vi "Digital Serial Configuration Popup.vi"() -> ()   [LabVIEW 2021, in "Audio Popup UI.lvlib"]
uses:
  Audio Popup UI.lvlib
  controls/digital audio protocol/digital audio protocol settings.ctl
  <vilib>/PDM Acquisition Toolkit/shared/controls/PCM Data Justification.ctl
  <vilib>/PDM Acquisition Toolkit/shared/controls/PCM Bit Endianness.ctl
  <vilib>/PDM Acquisition Toolkit/shared/controls/Digital Edge.ctl
  <vilib>/PDM Acquisition Toolkit/host/Classes/Session/Controls/Logic Levels.ctl
  <vilib>/PDM Acquisition Toolkit/shared/PDM Shared.lvlib
  <vilib>/PDM Acquisition Toolkit/host/Classes/Session/DecoderSession.lvclass
  controls/digital audio protocol/digital audio protocol controls.lvlib
panel:
  in  "channel 0 offset":u32=1
  in  "Save":bool
  in  "Configuration File":path
  in  "logic level":enum32{"3.3 V", "1.8 V", "1.2 V"}(ring) caption="Logic level"
  in  "master clock rate":dbl=12288000.0 caption="Master clock rate" format="%#_6pHz"
  out "Bit clock rate":dbl=3072000.0 format="%#_6pHz"
  in  "number of channels":u32=2 caption="Number of channels"
  in  "TDM":bool
  in  "RJ":bool
  in  "LJ":bool
  in  "I2S":bool
  in  "bit clock edge sync":enum32{"Rising", "Falling"}(ring)=enum."Falling" caption="Bit clock edge sync"
  in  "frame clock rate":dbl=48000.0 caption="Frame clock rate" format="%#_6pHz"
  in  "data justification":enum32{"Left Justified", "Right Justified"}(ring) caption="Data justification"
  in  "endianness":enum32{"MSB First", "LSB First"}(ring) caption="Endianness"
  in  "bit depth":u32=24 caption="Bit depth"
  in  "channel length":u32=32 caption="Channel length"
  in  "frame sync edge for channel 0":enum32{"Rising", "Falling"}(ring)=enum."Falling" caption="Frame sync edge for Channel 0"
  # "Audio Protocol"
  # "Clock Settings"
  # "Signal Level"
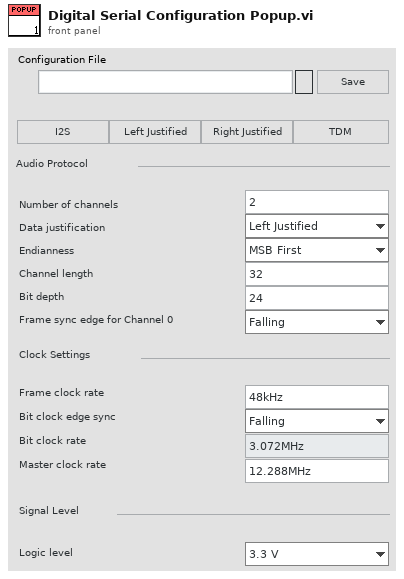
[diagram p1: front panel]
types:
  T1 = typedef "digital audio protocol controls.lvlib/digital audio protocol settings.ctl" = cluster{"number of channels":u32, "data justification":T2, "endianness":T3, "channel length":u32, "bit depth":u32, "frame clock rate":dbl, "bit clock edge sync":T4, "master clock rate":dbl, "Logic Level":T5, "frame sync edge for channel 0":T4, "Channel 0 Offset":u32}
  T2 = typedef "PDM Shared.lvlib/PCM Data Justification.ctl" = enum16{"Left Justified", "Right Justified"}
  T3 = typedef "PDM Shared.lvlib/PCM Bit Endianness.ctl" = enum16{"MSB First", "LSB First"}
  T4 = typedef "PDM Shared.lvlib/Digital Edge.ctl" = enum8{"Rising", "Falling"}
  T5 = typedef "PDM Acquisition Class Library.lvlib/DecoderSession.lvclass/Logic Levels.ctl" = enum16{"3.3 V", "1.8 V", "1.2 V"}
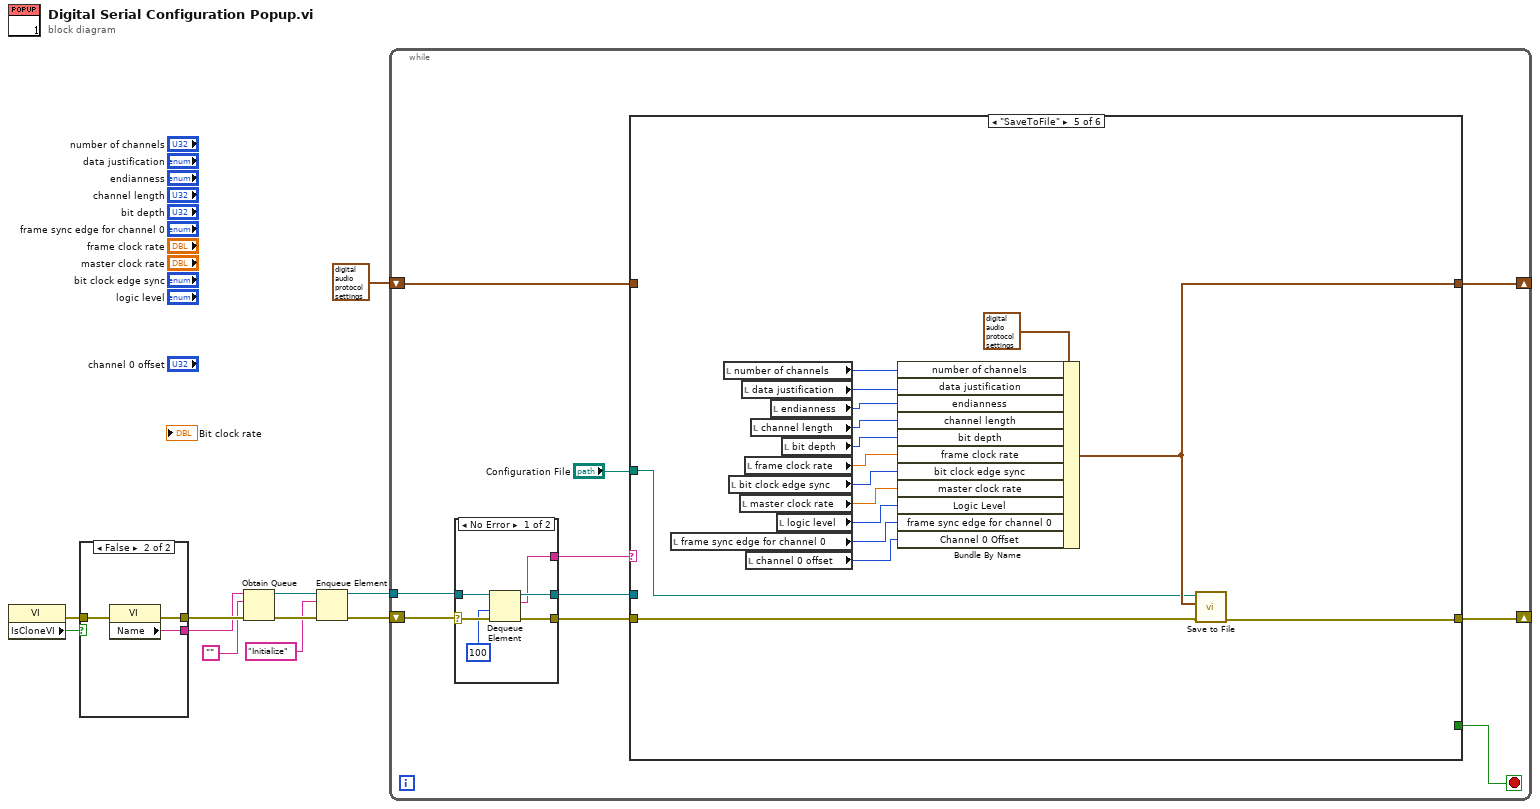
[diagram p0: block diagram]
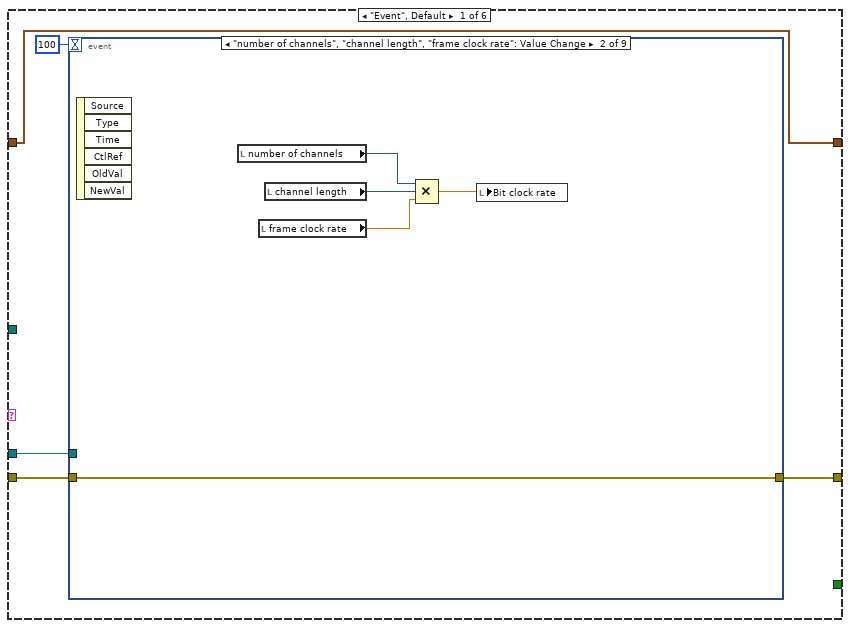
[diagram p2: hidden frame]
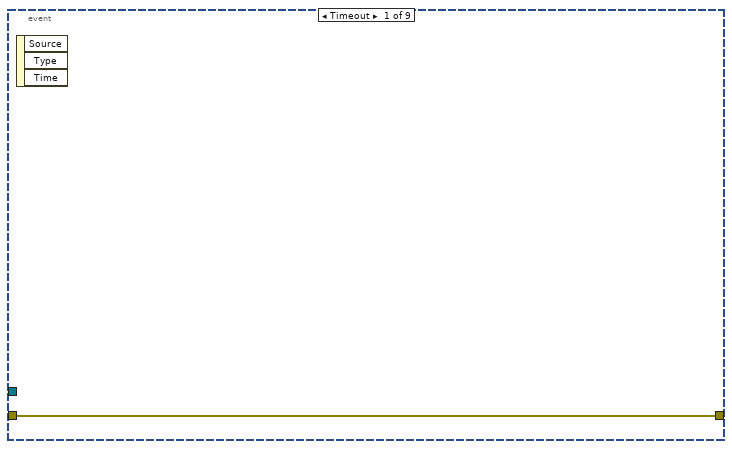
[diagram p3: hidden frame]
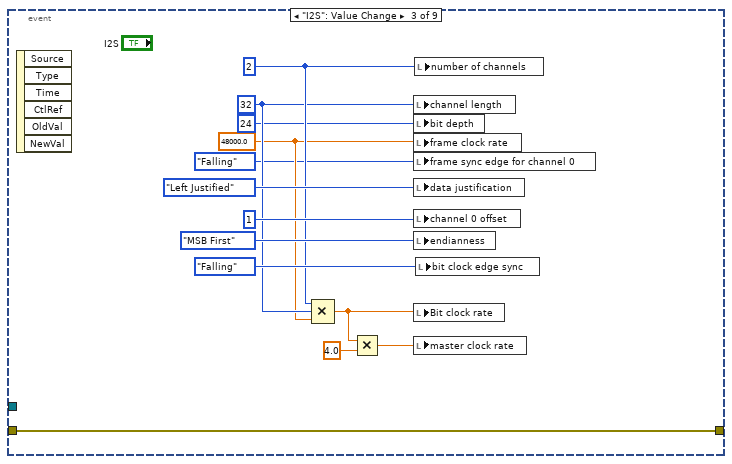
[diagram p4: hidden frame]
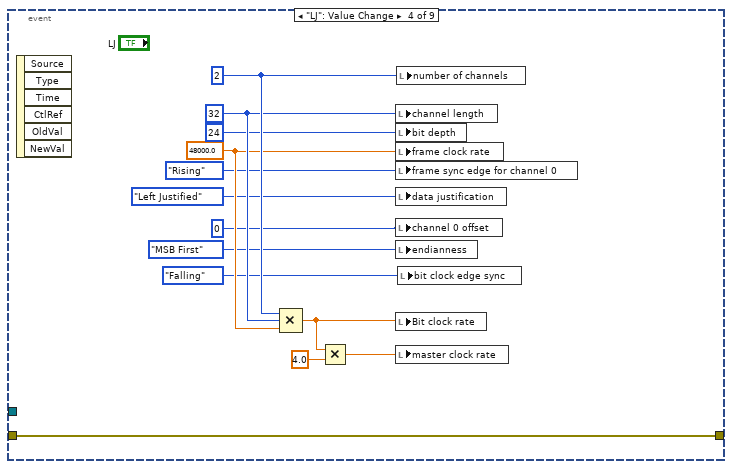
[diagram p5: hidden frame]
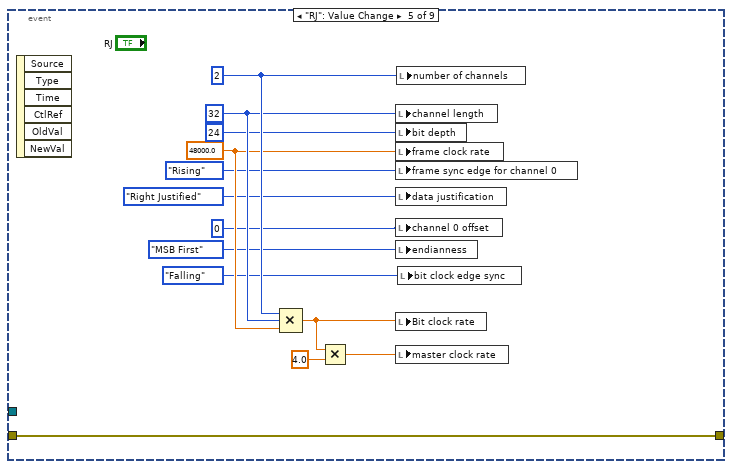
[diagram p6: hidden frame]
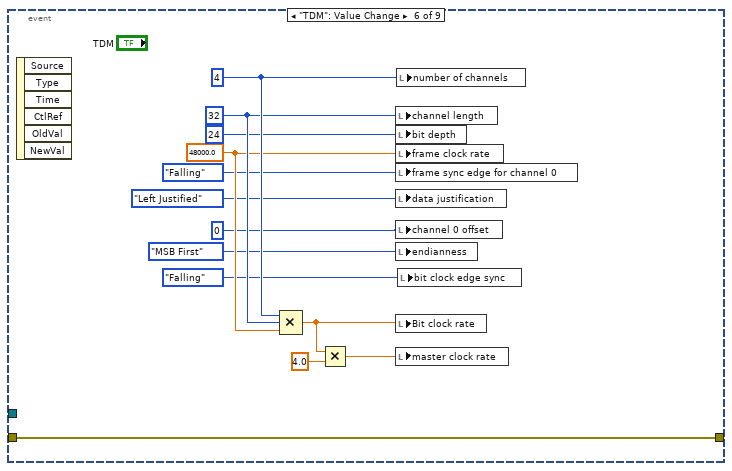
[diagram p7: hidden frame]
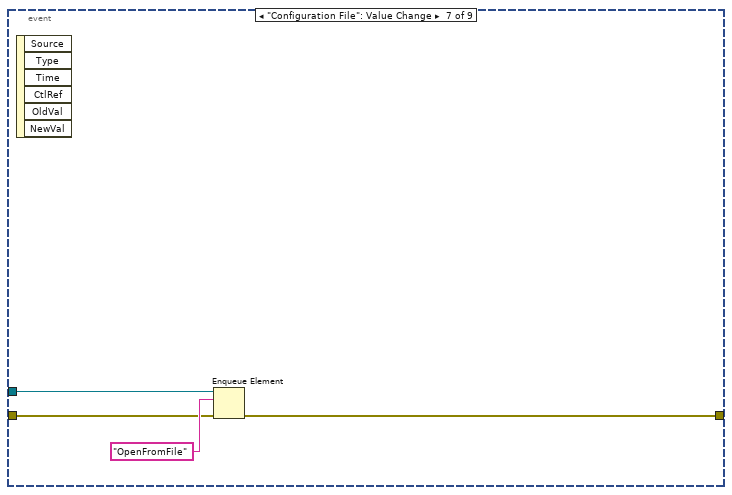
[diagram p8: hidden frame]
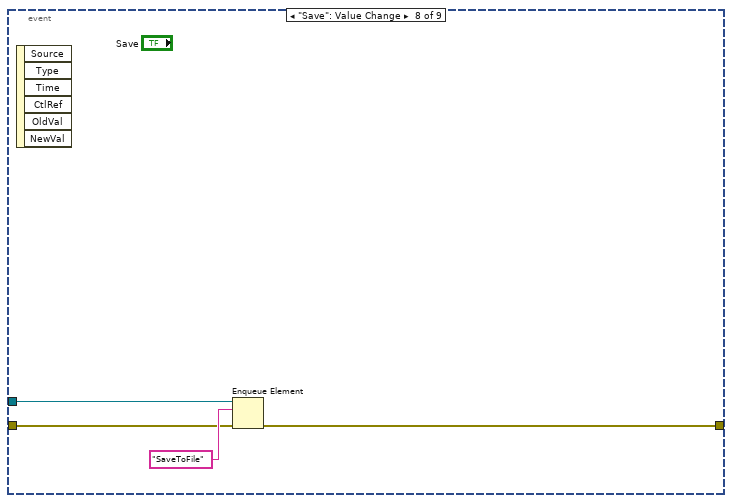
[diagram p9: hidden frame]
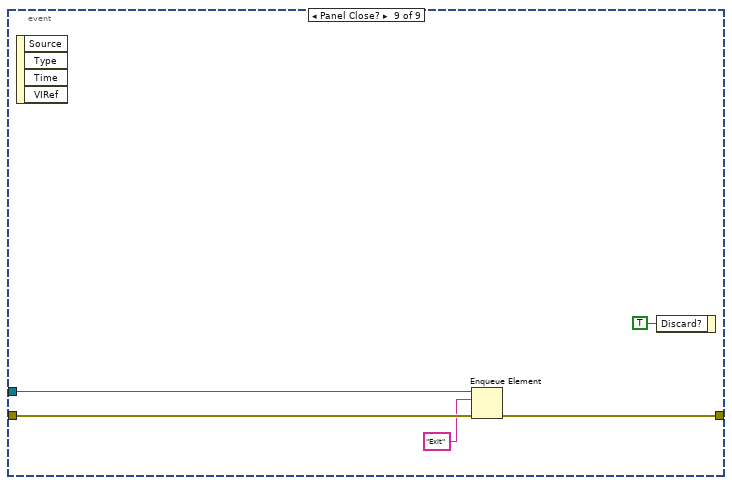
[diagram p10: hidden frame]
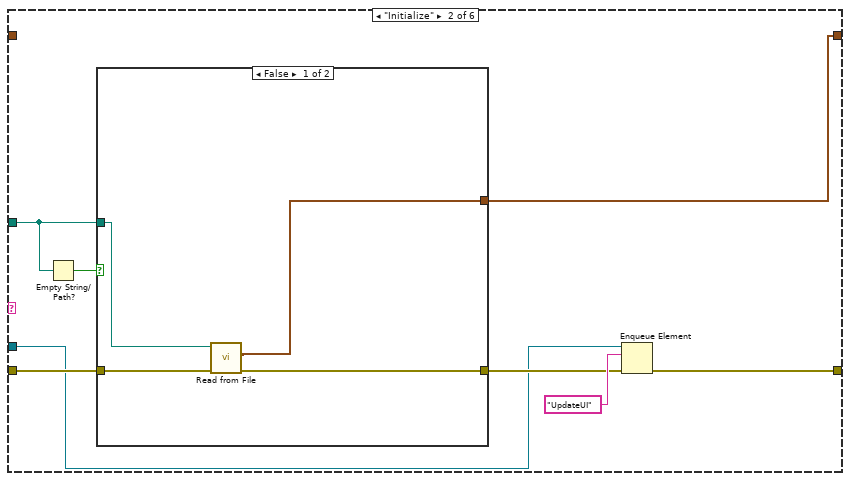
[diagram p11: hidden frame]
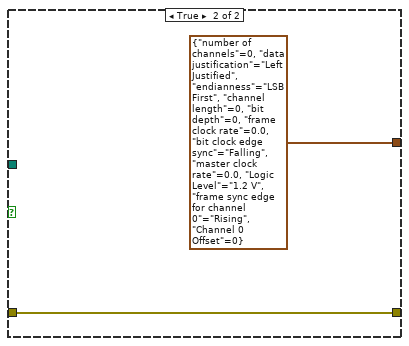
[diagram p12: hidden frame]
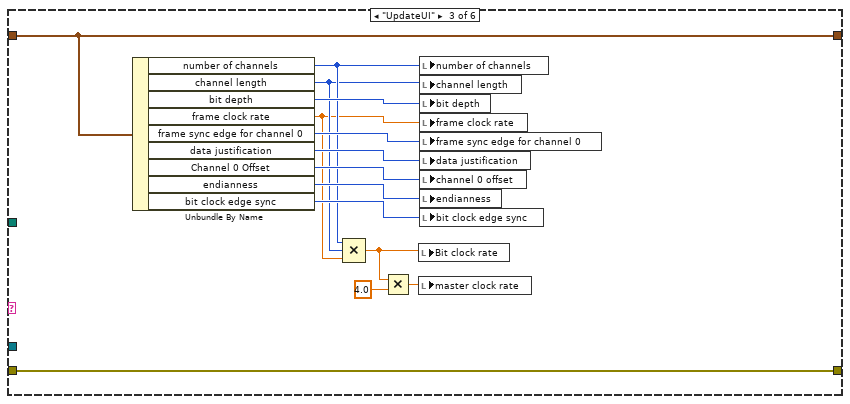
[diagram p13: hidden frame]
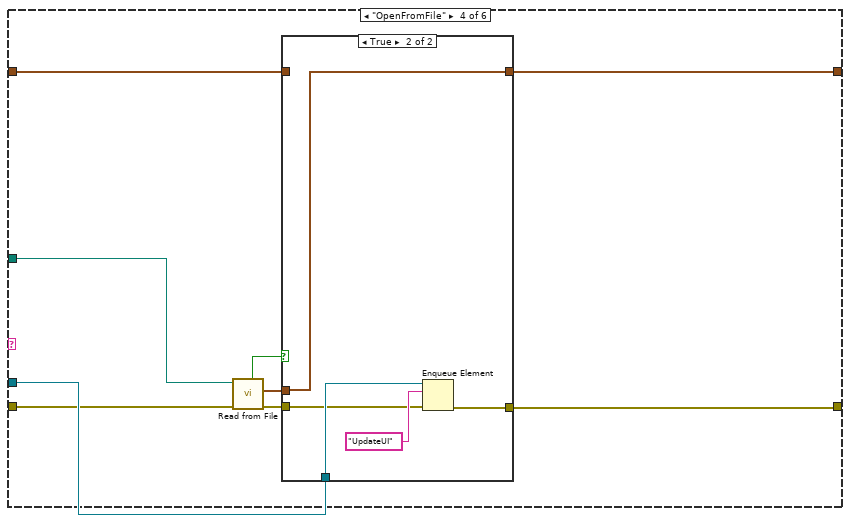
[diagram p14: hidden frame]
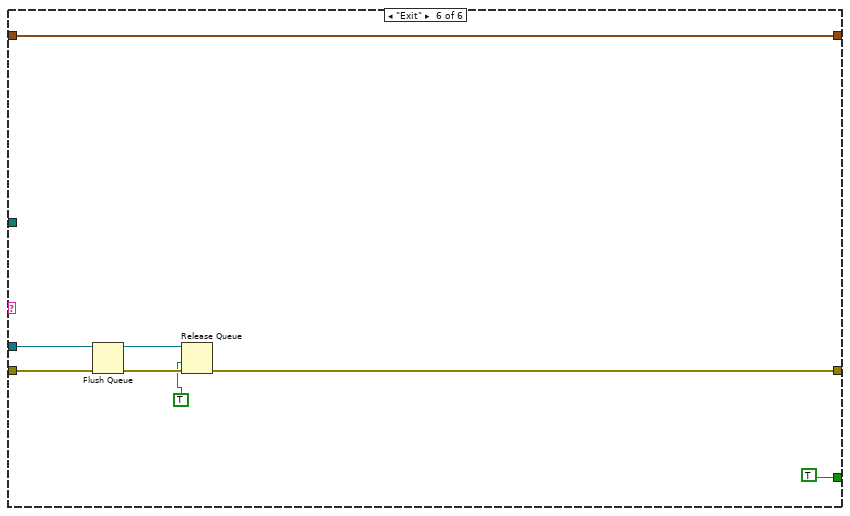
[diagram p16: hidden frame]
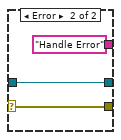
[diagram p17: hidden frame]
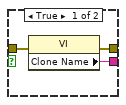
[diagram p18: hidden frame]
diagram:
  n1 = property class="VI"() -> (error out=w4:errorcluster, "IsCloneVI"=w5:bool)  [unwired: 2 in, 1 out]
  n2 = case shown="False" w5 {
    tunnel: [w14 w17] -> w11
    tunnel: [w13 w16] -> w10
    tunnel: w4 -> [w12 w15]
    frame True {
      n3 = property class="VI"(error in=w12) -> (error out=w14:errorcluster, "Clone Name"=w13:string)  [unwired: 1 in, 1 out]
    }
    frame False {
      n4 = property class="VI"(error in=w15) -> (error out=w17:errorcluster, "Name"=w16:string)  [unwired: 1 in, 1 out]
    }
  }
  n5 = Obtain Queue(name (unnamed)=w10, element data type="", error in (no error)=w11) -> (queue out=w8:refnum<queue>, error out=w9:errorcluster)  [unwired: 2 in, 1 out]
  n6 = Enqueue Element(queue=w8, element="Initialize", error in (no error)=w9) -> (queue out=w2:refnum<queue>, error out=w3:errorcluster)  [unwired: 1 in, 1 out]
  n7 = while {
    tunnel: w2 -> [w26]
    shift-right: [w22] -> _
    shift-left: w3 -> [w27]
    shift-right: [w19] -> _
    shift-left: T1 {"number of channels"=0, "data justification"=enum."Left Justified", "endianness"=enum."LSB First", "channel length"=0, "bit depth"=0, "frame clock rate"=0.0, "bit clock edge sync"=enum."Falling", "master clock rate"=0.0, "Logic Level"=enum."1.2 V", "frame sync edge for channel 0"=enum."Rising", "Channel 0 Offset"=0} ("digital audio protocol settings") -> [w20]
    stop <- w21 stop-if-true
    n8 = case shown="No Error" w27 {
      selector: w27 -> [w177 w180]
      tunnel: [w176 w180] -> w23
      tunnel: w26 -> [w175 w179]
      tunnel: [w174 w179] -> w24
      tunnel: [w173 "Handle Error"] -> w25
      frame No Error {
        n9 = Dequeue Element(queue=w175, timeout in ms (-1)=100, error in (no error)=w177) -> (queue out=w174:refnum<queue>, element=w173:string, error out=w176:errorcluster)  [unwired: 1 out]
      }
      frame Error {
      }
    }
    n10 = case shown="\"SaveToFile\"" w25 {
      tunnel: w24 -> [w30 w104 _ w140 _ w167]
      tunnel: w23 -> [w31 w111 w131 w137 w151 w168]
      tunnel: [w29 w105 w131 w139 w150 w165] -> w22
      tunnel: [_ _ _ _ _ TRUE] -> w21
      tunnel: w20 -> [w28 _ w130 w134 _ w164]
      tunnel: [w28 w108 w130 w133 w149 w164] -> w19
      tunnel: "Configuration File" -> [_ w109 _ w138 w148 _]
      frame "Event", Default {
        n11 = event shown="[1] \"number of channels\", \"channel length\", \"frame clock rate\": Value Change" {
          selector: _ -> [_ _ _ _ _ _ _ _ _]
          dyn-events: _ -> [_ _ _ _ _ _ _ _ _]
          timeout: 100 -> [_ _ _ _ _ _ _ _ _]
          tunnel: w31 -> [w33 w34 w39 w52 w65 w78 w93 w97 w102]
          tunnel: w30 -> [_ _ _ _ _ _ w92 w96 w101]
          tunnel: [w33 w34 w39 w52 w65 w78 w91 w95 w100] -> w29
          event Timeout {
            n12 = event-data() -> ()  [unwired: 1 in, 3 out]
          }
          event "number of channels", "channel length", "frame clock rate": Value Change {
            n13 = event-data() -> ()  [unwired: 1 in, 6 out]
            n14 = local read "number of channels"() -> (w36:u32)
            n15 = local read "frame clock rate"() -> (w35:dbl)
            n16 = local read "channel length"() -> (w37:u32)
            n17 = Compound Arithmetic op=MULTIPLY(w36, w37, w35) -> (w38:dbl)
            n18 = local write "Bit clock rate"(w38) -> ()
          }
          event "I2S": Value Change {
            w42 = 48000.0 ("Frame Clock Rate")
            w43 = u32 32 ("Channel Length")
            w44 = u32 2 ("Number of Channels")
            n19 = event-data() -> ()  [unwired: 1 in, 6 out]
            n20 = Compound Arithmetic op=MULTIPLY(w44, w43, w42) -> (w50:dbl)
            n21 = Multiply(x=w50, y=4.0) -> (x*y=w49:dbl)
            n22 = local write "channel length"(w43) -> ()
            n23 = local write "bit depth"(u32 24 ("Bit Depth")) -> ()
            n24 = local write "frame clock rate"(w42) -> ()
            n25 = local write "frame sync edge for channel 0"(enum32{"Rising", "Falling"}."Falling" ("bit clock edge sync")) -> ()
            n26 = local write "data justification"(enum32{"Left Justified", "Right Justified"}."Left Justified" ("data justification")) -> ()
            n27 = local write "channel 0 offset"(u32 1 ("Channel 0 Offset")) -> ()
            n28 = local write "endianness"(enum32{"MSB First", "LSB First"}."MSB First" ("endianness")) -> ()
            n29 = local write "Bit clock rate"(w50) -> ()
            n30 = local write "master clock rate"(w49) -> ()
            n31 = local write "number of channels"(w44) -> ()
            n32 = local write "bit clock edge sync"(enum32{"Rising", "Falling"}."Falling" ("frame sync edge for channel 0")) -> ()
          }
          event "LJ": Value Change {
            w60 = 48000.0 ("Frame Clock Rate")
            w62 = u32 32 ("Channel Length")
            w63 = u32 2 ("Number of Channels")
            n33 = event-data() -> ()  [unwired: 1 in, 6 out]
            n34 = Compound Arithmetic op=MULTIPLY(w63, w62, w60) -> (w54:dbl)
            n35 = Multiply(x=w54, y=4.0) -> (x*y=w53:dbl)
            n36 = local write "channel length"(w62) -> ()
            n37 = local write "bit depth"(u32 24 ("Bit Depth")) -> ()
            n38 = local write "frame clock rate"(w60) -> ()
            n39 = local write "frame sync edge for channel 0"(enum32{"Rising", "Falling"}."Rising" ("bit clock edge sync")) -> ()
            n40 = local write "data justification"(enum32{"Left Justified", "Right Justified"}."Left Justified" ("data justification")) -> ()
            n41 = local write "channel 0 offset"(u32 0 ("Channel 0 Offset")) -> ()
            n42 = local write "endianness"(enum32{"MSB First", "LSB First"}."MSB First" ("endianness")) -> ()
            n43 = local write "Bit clock rate"(w54) -> ()
            n44 = local write "master clock rate"(w53) -> ()
            n45 = local write "number of channels"(w63) -> ()
            n46 = local write "bit clock edge sync"(enum32{"Rising", "Falling"}."Falling" ("frame sync edge for channel 0")) -> ()
          }
          event "RJ": Value Change {
            w73 = 48000.0 ("Frame Clock Rate")
            w75 = u32 32 ("Channel Length")
            w76 = u32 2 ("Number of Channels")
            n47 = event-data() -> ()  [unwired: 1 in, 6 out]
            n48 = Compound Arithmetic op=MULTIPLY(w76, w75, w73) -> (w67:dbl)
            n49 = Multiply(x=w67, y=4.0) -> (x*y=w66:dbl)
            n50 = local write "channel length"(w75) -> ()
            n51 = local write "bit depth"(u32 24 ("Bit Depth")) -> ()
            n52 = local write "frame clock rate"(w73) -> ()
            n53 = local write "frame sync edge for channel 0"(enum32{"Rising", "Falling"}."Rising" ("bit clock edge sync")) -> ()
            n54 = local write "data justification"(enum32{"Left Justified", "Right Justified"}."Right Justified" ("data justification")) -> ()
            n55 = local write "channel 0 offset"(u32 0 ("Channel 0 Offset")) -> ()
            n56 = local write "endianness"(enum32{"MSB First", "LSB First"}."MSB First" ("endianness")) -> ()
            n57 = local write "Bit clock rate"(w67) -> ()
            n58 = local write "master clock rate"(w66) -> ()
            n59 = local write "number of channels"(w76) -> ()
            n60 = local write "bit clock edge sync"(enum32{"Rising", "Falling"}."Falling" ("frame sync edge for channel 0")) -> ()
          }
          event "TDM": Value Change {
            w86 = 48000.0 ("Frame Clock Rate")
            w88 = u32 32 ("Channel Length")
            w89 = u32 4 ("Number of Channels")
            n61 = event-data() -> ()  [unwired: 1 in, 6 out]
            n62 = Compound Arithmetic op=MULTIPLY(w89, w88, w86) -> (w80:dbl)
            n63 = Multiply(x=w80, y=4.0) -> (x*y=w79:dbl)
            n64 = local write "channel length"(w88) -> ()
            n65 = local write "bit depth"(u32 24 ("Bit Depth")) -> ()
            n66 = local write "frame clock rate"(w86) -> ()
            n67 = local write "frame sync edge for channel 0"(enum32{"Rising", "Falling"}."Falling" ("bit clock edge sync")) -> ()
            n68 = local write "data justification"(enum32{"Left Justified", "Right Justified"}."Left Justified" ("data justification")) -> ()
            n69 = local write "channel 0 offset"(u32 0 ("Channel 0 Offset")) -> ()
            n70 = local write "endianness"(enum32{"MSB First", "LSB First"}."MSB First" ("endianness")) -> ()
            n71 = local write "Bit clock rate"(w80) -> ()
            n72 = local write "master clock rate"(w79) -> ()
            n73 = local write "number of channels"(w89) -> ()
            n74 = local write "bit clock edge sync"(enum32{"Rising", "Falling"}."Falling" ("frame sync edge for channel 0")) -> ()
          }
          event "Configuration File": Value Change {
            n75 = event-data() -> ()  [unwired: 1 in, 6 out]
            n76 = Enqueue Element(queue=w92, element="OpenFromFile", error in (no error)=w93) -> (error out=w91:errorcluster)  [unwired: 1 in, 2 out]
          }
          event "Save": Value Change {
            n77 = event-data() -> ()  [unwired: 1 in, 6 out]
            n78 = Enqueue Element(queue=w96, element="SaveToFile", error in (no error)=w97) -> (error out=w95:errorcluster)  [unwired: 1 in, 2 out]
          }
          event Panel Close? {
            n79 = event-data() -> ()  [unwired: 1 in, 4 out]
            n80 = Enqueue Element(queue=w101, element="Exit", error in (no error)=w102) -> (error out=w100:errorcluster)  [unwired: 1 in, 2 out]
            n81 = event-data("Discard?"=TRUE) -> ()  [unwired: 1 in, 1 out]
          }
        }
      }
      frame "Initialize" {
        n82 = Empty String/Path?(string/path=w109) -> (empty?=w110:bool)
        n83 = case shown="False" w110 {
          tunnel: w111 -> [w115 w116]
          tunnel: w109 -> [w114 _]
          tunnel: [w112 T1 {"number of channels"=0, "data justification"=enum."Left Justified", "endianness"=enum."LSB First", "channel length"=0, "bit depth"=0, "frame clock rate"=0.0, "bit clock edge sync"=enum."Falling", "master clock rate"=0.0, "Logic Level"=enum."1.2 V", "frame sync edge for channel 0"=enum."Rising", "Channel 0 Offset"=0} ("digital audio protocol settings")] -> w108
          tunnel: [w113 w116] -> w106
          frame False {
            n84 = call "Read from File.vi"("error in (no error)"=w115, "file path"=w114) -> ("error out"=w113:errorcluster, "digital audio protocol settings"=w112:T1)  [unwired: 7 in, 1 out]
          }
          frame True {
          }
        }
        n85 = Enqueue Element(queue=w104, element="UpdateUI", error in (no error)=w106) -> (error out=w105:errorcluster)  [unwired: 1 in, 2 out]
      }
      frame "UpdateUI" {
        n86 = Unbundle By Name(w130) -> ("number of channels"=w121:u32, "channel length"=w120:u32, "bit depth"=w129:u32, "frame clock rate"=w119:dbl, "frame sync edge for channel 0"=w128:T4, "data justification"=w127:T2, "Channel 0 Offset"=w126:u32, "endianness"=w125:T3, "bit clock edge sync"=w124:T4)
        n87 = Compound Arithmetic op=MULTIPLY(w121, w120, w119) -> (w118:dbl)
        n88 = Multiply(x=w118, y=4.0) -> (x*y=w122:dbl)
        n89 = local write "Bit clock rate"(w118) -> ()
        n90 = local write "master clock rate"(w122) -> ()
        n91 = local write "number of channels"(w121) -> ()
        n92 = local write "channel length"(w120) -> ()
        n93 = local write "bit depth"(w129) -> ()
        n94 = local write "frame clock rate"(w119) -> ()
        n95 = local write "frame sync edge for channel 0"(w128) -> ()
        n96 = local write "data justification"(w127) -> ()
        n97 = local write "channel 0 offset"(w126) -> ()
        n98 = local write "endianness"(w125) -> ()
        n99 = local write "bit clock edge sync"(w124) -> ()
      }
      frame "OpenFromFile" {
        n100 = call "Read from File.vi"("error in (no error)"=w137, "file path"=w138) -> ("error out"=w136:errorcluster, "digital audio protocol settings"=w132:T1, "file exists?"=w135:bool)  [unwired: 7 in]
        n101 = case shown="True" w135 {
          tunnel: w140 -> [_ w146]
          tunnel: [w141 w145] -> w139
          tunnel: w136 -> [w141 w144]
          tunnel: w134 -> [w142 _]
          tunnel: [w142 w143] -> w133
          tunnel: w132 -> [_ w143]
          frame False {
          }
          frame True {
            n102 = Enqueue Element(queue=w146, element="UpdateUI", error in (no error)=w144) -> (error out=w145:errorcluster)  [unwired: 1 in, 2 out]
          }
        }
      }
      frame "SaveToFile" {
        n103 = local read "frame sync edge for channel 0"() -> (w153:enum32{"Rising", "Falling"})
        n104 = local read "number of channels"() -> (w162:u32)
        n105 = local read "bit clock edge sync"() -> (w156:enum32{"Rising", "Falling"})
        n106 = local read "master clock rate"() -> (w155:dbl)
        n107 = local read "data justification"() -> (w161:enum32{"Left Justified", "Right Justified"})
        n108 = local read "frame clock rate"() -> (w157:dbl)
        n109 = local read "channel 0 offset"() -> (w152:u32)
        n110 = local read "channel length"() -> (w159:u32)
        n111 = local read "endianness"() -> (w160:enum32{"MSB First", "LSB First"})
        n112 = local read "logic level"() -> (w154:enum32{"3.3 V", "1.8 V", "1.2 V"})
        n113 = local read "bit depth"() -> (w158:u32)
        n114 = Bundle By Name(cluster=T1 {"number of channels"=0, "data justification"=enum."Left Justified", "endianness"=enum."LSB First", "channel length"=0, "bit depth"=0, "frame clock rate"=0.0, "bit clock edge sync"=enum."Falling", "master clock rate"=0.0, "Logic Level"=enum."1.2 V", "frame sync edge for channel 0"=enum."Rising", "Channel 0 Offset"=0} ("input cluster"), "number of channels"=w162, "data justification"=w161, "endianness"=w160, "channel length"=w159, "bit depth"=w158, "frame clock rate"=w157, "bit clock edge sync"=w156, "master clock rate"=w155, "Logic Level"=w154, "frame sync edge for channel 0"=w153, "Channel 0 Offset"=w152) -> (w149:T1)
        n115 = call "Save to File.vi"("error in (no error)"=w151, "digital audio protocol settings"=w149, "file path"=w148) -> ("error out"=w150:errorcluster)  [unwired: 8 in]
      }
      frame "Exit" {
        n116 = Flush Queue(queue=w167, error in (no error)=w168) -> (queue out=w171:refnum<queue>, error out=w170:errorcluster)  [unwired: 1 out]
        n117 = Release Queue(queue=w171, force destroy? (F)=TRUE, error in (no error)=w170) -> (error out=w165:errorcluster)  [unwired: 2 out]
      }
    }
  }
